vi "Welcome.vi"() -> ()   [LabVIEW 2018]
uses:
  UI/UI.lvclass
  UI/UI.lvclass/UI.ctl
  UI/setEmbeddedVI.vi
  UI/setUIData.vi
panel:
  in  "Stop":bool
  in  "Melhores Pontuações":bool
  in  "Histórico de Partidas":bool
  in  "Informações do App":bool
  in  "Instruções":bool
  in  "Novo Jogo":bool
  in  "UI in":refnum<class "UI.lvclass">
  out "UI out":refnum<class "UI.lvclass">
  in  "error in (no error)":errorcluster
  out "error out":errorcluster
  # "Bem Vindo!!"
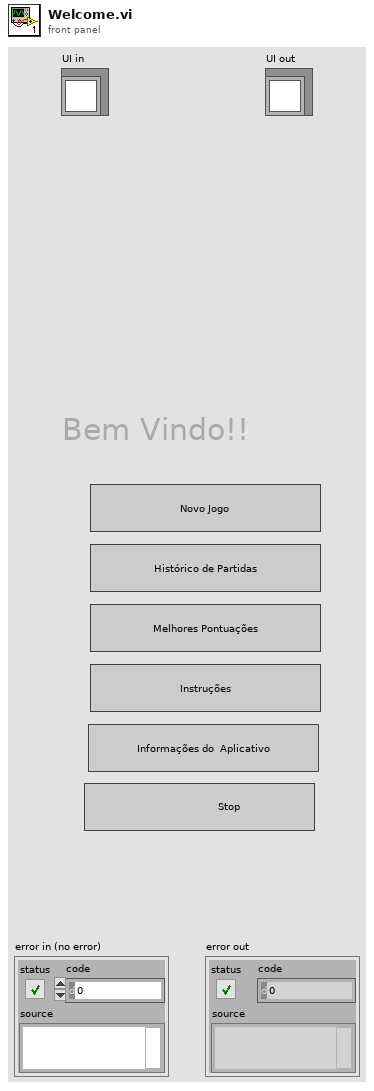
[diagram p1: front panel]
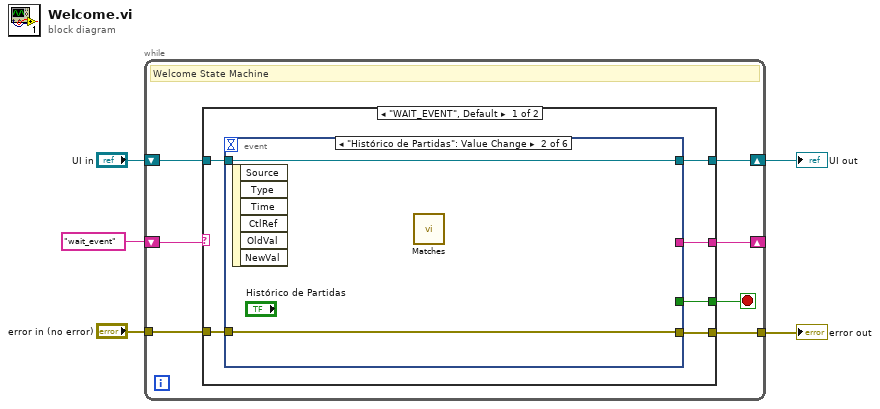
[diagram p0: block diagram]
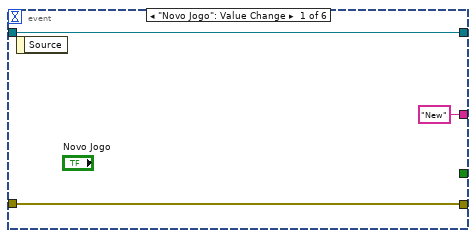
[diagram p2: hidden frame]
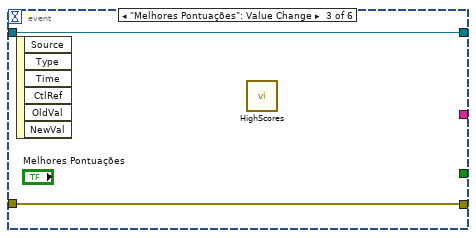
[diagram p3: hidden frame]
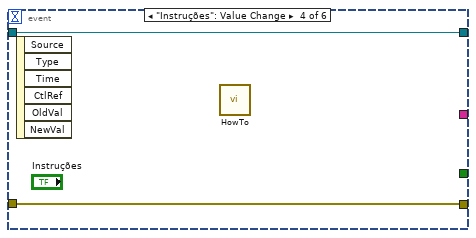
[diagram p4: hidden frame]
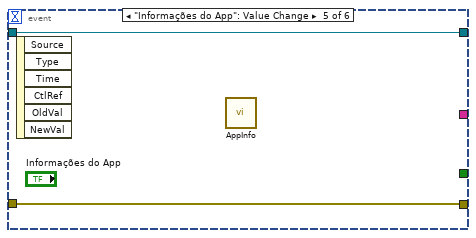
[diagram p5: hidden frame]
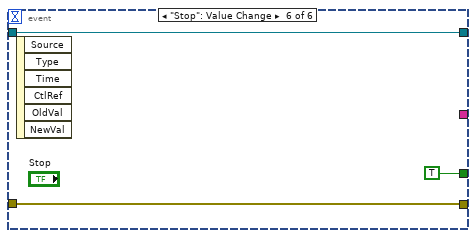
[diagram p6: hidden frame]
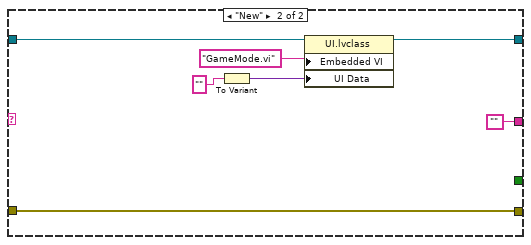
[diagram p7: hidden frame]
diagram:
  n1 = while {
    shift-right: [w11] -> w2
    shift-left: "UI in" -> [w12]
    tunnel: [w10] -> w4
    tunnel: "error in (no error)" -> [w9]
    shift-right: [w8] -> _
    shift-left: "wait_event" -> [w7]
    stop <- w6 stop-if-true
    # "Welcome State Machine"
    n2 = case shown="\"WAIT_EVENT\", Default" w7 {
      tunnel: w12 -> [w18 w36]
      tunnel: [w17 w35] -> w11
      tunnel: [w16 w39] -> w10
      tunnel: w9 -> [w15 w39]
      tunnel: [w14 ""] -> w8
      tunnel: [w13 _] -> w6
      frame "WAIT_EVENT", Default {
        n3 = event shown="[1] \"Histórico de Partidas\": Value Change" {
          selector: _ -> [_ _ _ _ _ _]
          dyn-events: _ -> [_ _ _ _ _ _]
          timeout: _ -> [_ _ _ _ _ _]
          tunnel: [w21 w23 w25 w27 w29 w32] -> w17
          tunnel: w18 -> [w21 w23 w25 w27 w29 w32]
          tunnel: [w20 w22 w24 w26 w28 w31] -> w16
          tunnel: w15 -> [w20 w22 w24 w26 w28 w31]
          tunnel: ["New" _ _ _ _ _] -> w14
          tunnel: [_ _ _ _ _ TRUE] -> w13
          event "Novo Jogo": Value Change {
            n4 = event-data() -> ()  [unwired: 1 in, 1 out]
          }
          event "Histórico de Partidas": Value Change {
            n5 = event-data() -> ()  [unwired: 1 in, 6 out]
            n6 = call "Matches.vi"() -> ()  [unwired: 12 in]
          }
          event "Melhores Pontuações": Value Change {
            n7 = event-data() -> ()  [unwired: 1 in, 6 out]
            n8 = call "HighScores.vi"() -> ()  [unwired: 12 in]
          }
          event "Instruções": Value Change {
            n9 = event-data() -> ()  [unwired: 1 in, 6 out]
            n10 = call "HowTo.vi"() -> ()  [unwired: 12 in]
          }
          event "Informações do App": Value Change {
            n11 = event-data() -> ()  [unwired: 1 in, 6 out]
            n12 = call "AppInfo.vi"() -> ()  [unwired: 12 in]
          }
          event "Stop": Value Change {
            n13 = event-data() -> ()  [unwired: 1 in, 6 out]
          }
        }
      }
      frame "New" {
        n14 = To Variant(anything="") -> (Variant=w38:variant)
        n15 = property class="UI.lvclass"(reference=w36, "Embedded VI"="GameMode.vi" ("String <Replace Me>"), "UI Data"=w38) -> (reference out=w35:refnum<class "UI.lvclass">)  [unwired: 1 in, 1 out]
      }
    }
  }
  "UI out" <- w2
  "error out" <- w4
